vi "CopyClass.vi"(8 "error in (no error)":errorcluster, 9 "Actor Method VI Name":string, 10 "Subfolders":string, 11 "CS++Actor in":refnum<class "CS++Actor.lvclass">) -> (0 "error out":errorcluster, 1 "New Class Path":path, 2 "AddItemFromMemory":refnum<vi>, 3 "CS++Actor out":refnum<class "CS++Actor.lvclass">)   [LabVIEW 2014, in "CS++Actor.lvlib" / "CS++Actor.lvclass"]
doc: "Copies the template to the location of the new message class."
uses:
  CS++Actor.lvclass
  CS++Actor.lvclass/CS++Actor.ctl
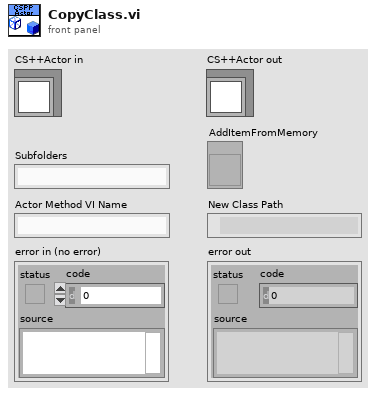
[diagram p1: front panel]
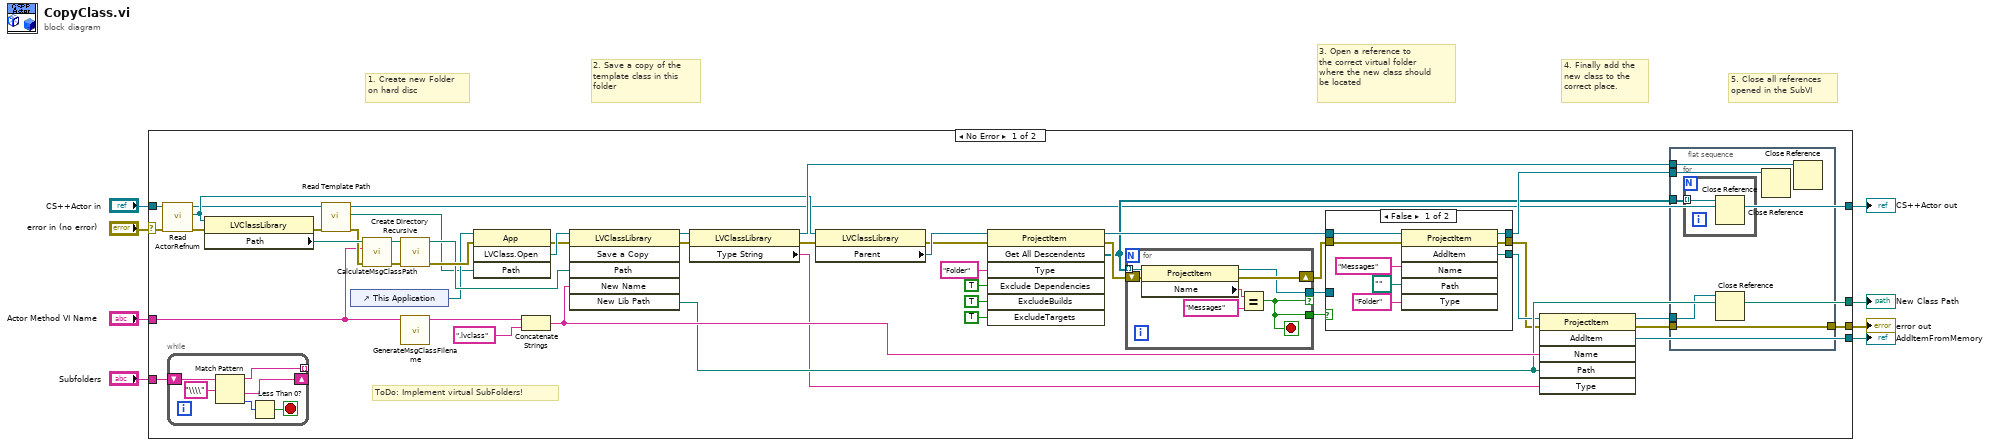
[diagram p0: block diagram]
diagram:
  # "5. Close all references\nopened in the SubVI"
  # "4. Finally add the\nnew class to the\ncorrect place."
  # "3. Open a reference to\nthe correct virtual folder\nwhere the new class should\nbe located"
  # "2. Save a copy of the\ntemplate class in this \nfolder"
  # "1. Create new Folder\non hard disc"
  n1 = case shown="No Error" "error in (no error)" {
    selector: "error in (no error)" -> [w43 w87]
    tunnel: [w51 _] -> w8
    tunnel: "Actor Method VI Name" -> [w10 _]
    tunnel: [w19 w87] -> w6
    tunnel: [w46 _] -> w4
    tunnel: [w13 w86] -> w3
    tunnel: "CS++Actor in" -> [w44 w86]
    tunnel: "Subfolders" -> [w11 _]
    frame No Error {
      # "ToDo: Implement virtual SubFolders!"
      n2 = call "Read ActorRefnum.vi"("error in (no error)"=w43, "CS++Actor in"=w44) -> ("error out"=w42:errorcluster, "ActorRefnum"=w34:refnum<vi>, "CS++Actor out"=w14:refnum<class "CS++Actor.lvclass">)  [unwired: 7 in]
      n3 = while {
        shift-right: [w59] -> _
        shift-left: w11 -> [w61]
        tunnel: [w58] -> _ mode=indexing
        stop <- w57 stop-if-true
        n4 = Match Pattern(string=w61, regular expression="\\\\") -> (before substring=w58:string, after substring=w59:string, offset past match=w56:i32)  [unwired: 1 in, 1 out]
        n5 = Less Than 0?(x=w56) -> (x < 0?=w57:bool)
      }
      n6 = property class="LVClassLibrary"(reference=w34, error in=w42) -> (error out=w16:errorcluster, "Path"=w41:path)  [unwired: 1 out]
      n7 = call "Read Template Path.vi"("error in (no error)"=w16, "CS++Actor in"=w14) -> ("error out"=w15:errorcluster, "Template Path"=w12:path, "CS++Actor out"=w13:refnum<class "CS++Actor.lvclass">)  [unwired: 7 in]
      n8 = control-ref of="This Application"() -> (w36:refnum<vi>)
      n9 = call "CalculateMsgClassPath.vi"("error in (no error)"=w15, "Method VI Name"=w10, "Actor Class Path"=w41) -> ("error out"=w40:errorcluster, "Message Class Path"=w39:path)  [unwired: 7 in]
      n10 = call <vilib>:"Create Directory Recursive.vi"("error in (no error)"=w40, "directory"=w39) -> ("error out"=w38:errorcluster, "directory copy"=w37:path)  [unwired: 3 in, 1 out]
      n11 = call "GenerateMsgClassFilename.vi"("Target Method"=w10) -> ("Msg Class File Name"=w9:string)  [unwired: 10 in]
      n12 = invoke class="App" method="LVClass.Open"(reference=w36, error in=w38, "Path"=w12) -> (error out=w54:errorcluster, "LVClass.Open"=w55:refnum<vi>)  [unwired: 1 in, 2 out]
      n13 = Concatenate Strings(w9, ".lvclass" ("regular expression")) -> (w52:string)
      n14 = invoke class="LVClassLibrary" method="Save a Copy"(reference=w55, error in=w54, "Path"=w37, "New Name"=w52) -> (reference out=w49:refnum<vi>, error out=w47:errorcluster, "New Lib Path"=w51:path)  [unwired: 2 in, 3 out]
      n15 = property class="LVClassLibrary"(reference=w49, error in=w47) -> (reference out=w48:refnum<vi>, error out=w35:errorcluster, "Type String"=w50:string)
      n16 = property class="LVClassLibrary"(reference=w34, error in=w35) -> (error out=w30:errorcluster, "Parent"=w32:refnum<vi>)  [unwired: 1 out]
      n17 = invoke class="ProjectItem" method="Get All Descendents"(reference=w32, error in=w30, "Type"="Folder", "Exclude Dependencies"=TRUE ("ExcludeDependencies"), "ExcludeBuilds"=TRUE, "ExcludeTargets"=TRUE) -> (reference out=w31:refnum<vi>, error out=w25:errorcluster, "All Descendents"=w20:refnum<vi>[])  [unwired: 1 in, 4 out]
      n18 = for {
        tunnel: w20 -> [w85] mode=indexing
        shift-right: [w83] -> w23
        shift-left: w25 -> [w84]
        tunnel: [w80] -> w22 if=w79
        tunnel: [w79] -> w24
        stop <- w79 stop-if-true
        n19 = property class="ProjectItem"(reference=w85, error in=w84) -> (reference out=w80:refnum<vi>, error out=w83:errorcluster, "Name"=w82:string)
        n20 = Equal?(x=w82, y="Messages") -> (x = y?=w79:bool)
      }
      n21 = case shown="False" w24 {
        tunnel: [w73 w78] -> w45
        tunnel: [w71 w77] -> w33
        tunnel: w31 -> [w70 w76]
        tunnel: w23 -> [w69 w77]
        tunnel: w22 -> [_ w78]
        tunnel: [w68 w76] -> w21
        frame False {
          n22 = invoke class="ProjectItem" method="AddItem"(reference=w70, error in=w69, "Name"="Messages", "Path"=path "", "Type"="Folder") -> (reference out=w68:refnum<vi>, error out=w71:errorcluster, "AddItem"=w73:refnum<vi>)  [unwired: 1 in, 3 out]
        }
        frame True {
        }
      }
      n23 = invoke class="ProjectItem" method="AddItem"(reference=w45, error in=w33, "Name"=w52, "Path"=w51, "Type"=w50) -> (reference out=w17:refnum<vi>, error out=w18:errorcluster, "AddItem"=w46:refnum<vi>)  [unwired: 1 in, 3 out]
      n24 = flat-sequence {
        tunnel: w48 -> [w66]
        tunnel: w21 -> [w65]
        tunnel: w20 -> [w64]
        tunnel: [w63] -> w19
        tunnel: w18 -> [w63]
        tunnel: w17 -> [w62]
        frame #0 {
          n25 = for {
            tunnel: w64 -> [w67] mode=indexing
            n26 = Close Reference(reference=w67) -> ()  [unwired: 1 in, 1 out]
          }
          n27 = Close Reference(reference=w62) -> ()  [unwired: 1 in, 1 out]
          n28 = Close Reference(reference=w65) -> ()  [unwired: 1 in, 1 out]
          n29 = Close Reference(reference=w66) -> ()  [unwired: 1 in, 1 out]
        }
      }
    }
    frame Error {
    }
  }
  "error out" <- w6
  "New Class Path" <- w8
  "AddItemFromMemory" <- w4
  "CS++Actor out" <- w3
